vi "ps.vi"() -> ()   [LabVIEW 2015]
panel:
  out "VISA resource name out 2":refnum<visa-resource-name>
  out "read buffer":string
  out "return count 2":u32
  out "error out 2":errorcluster
  in  "byte count":u32
  in  "Limit (A)":dbl
  out "Commands":string
  in  "Voltage (V)":dbl
  out "return count":u32
  in  "VISA resource name":refnum<visa-resource-name>
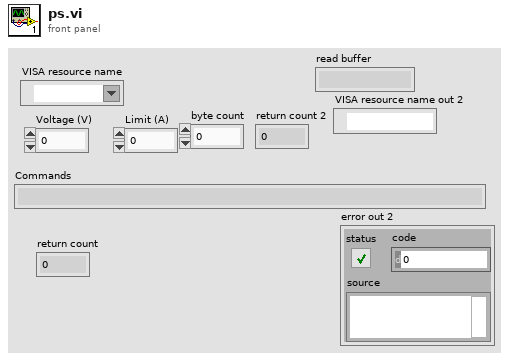
[diagram p1: front panel]
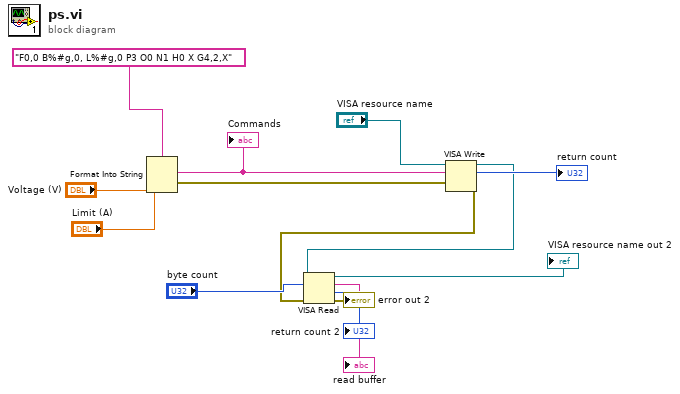
[diagram p0: block diagram]
diagram:
  n1 = Format Into String(format string="F0,0 B%#g,0, L%#g,0 P3 O0 N1 H0 X G4,2,X" ("F0,0X B%f,0,X L%f,0X P3X O0X"), "Voltage (V)", "Limit (A)") -> (resulting string=w10:string, error out=w11:errorcluster)  [unwired: 2 in]
  "Commands" <- w10
  n2 = VISA Write(VISA resource name="VISA resource name", write buffer=w10, error in (no error)=w11) -> (VISA resource name out=w1:refnum<visa-resource-name>, return count=→"return count":u32, error out=w2:errorcluster)
  n3 = VISA Read(VISA resource name=w1, byte count="byte count", error in (no error)=w2) -> (VISA resource name out=→"VISA resource name out 2":refnum<visa-resource-name>, read buffer=→"read buffer":string, return count=→"return count 2":u32, error out=→"error out 2":errorcluster)
